vi "showLUT.vi"(0 "Palette 2":cluster{u8, u8, u8}[](array[cluster]), 1 "Palette1":cluster{u8, u8, u8}[](array[cluster])) -> ()   [LabVIEW 2013]
uses:
  <vilib>/Analysis/1siggen.llb/Ramp Pattern by Samples.vi
  <vilib>/Analysis/NI_AALBase.lvlib
panel:
  in  "LUT 2":T1(ring)=enum."cold/hot (1/4)"
  in  "LUT1":T1(ring)=enum."cold/hot (1/4)"
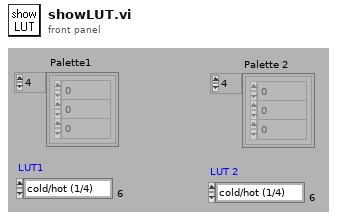
[diagram p1: front panel]
types:
  T1 = enum16{"gray", "gray + high", "gray + bounds", "gradient", "temperature", "cold/hot (1/2)", "cold/hot (1/4)", "odd/even"}
  T2 = enum32{"8 bits", "16 bits", "Float", "Complex", "RGB Chunky", "Compressed"}
  T3 = typedef "IMAQ Image.ctl" = refnum<image>
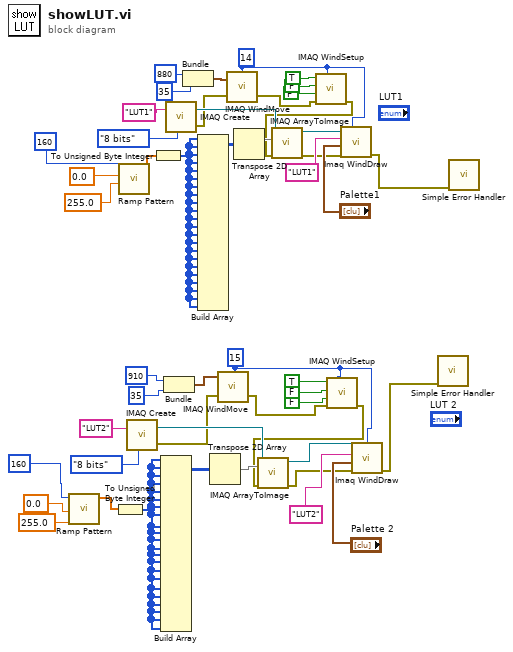
[diagram p0: block diagram]
diagram:
  w26 = 15 ("Window Number (0...15)")
  w35 = 14 ("Window Number (0...15)")
  n1 = call-poly <vilib>:"Ramp Pattern.vi"("start"=255.0, "end"=0.0, "samples"=160) -> ("Ramp Pattern"=w19:dbl[])  [unwired: 7 in, 1 out]
  n2 = To Unsigned Byte Integer(number=w19) -> (unsigned 8bit integer=w15:u8[])
  n3 = call-poly <vilib>:"Ramp Pattern.vi"("start"=255.0, "end"=0.0, "samples"=160) -> ("Ramp Pattern"=w50:dbl[])  [unwired: 7 in, 1 out]
  n4 = call "IMAQ Create"("Image Name"="LUT2", "Image Type"=T2."8 bits") -> ("New Image"=w24:T3, "error out"=w10:errorcluster)  [unwired: 2 in, 1 out]
  n5 = To Unsigned Byte Integer(number=w50) -> (unsigned 8bit integer=w34:u8[])
  n6 = Build Array(w15, w15, w15, w15, w15, w15, w15, w15, w15, w15, w15, w15, w15, w15, w15, w15, w15, w15, w15, w15, w15, w15) -> (w22:u8[][])
  n7 = Bundle(910, 35) -> (w30:cluster{i32, i32})  [unwired: 1 out]
  n8 = call "IMAQ Create"("Image Name"="LUT1", "Image Type"=T2."8 bits") -> ("New Image"=w49:T3, "error out"=w6:errorcluster)  [unwired: 2 in, 1 out]
  n9 = Bundle(880, 35) -> (w45:cluster{i32, i32})  [unwired: 1 out]
  n10 = Build Array(w34, w34, w34, w34, w34, w34, w34, w34, w34, w34, w34, w34, w34, w34, w34, w34, w34, w34, w34, w34, w34, w34) -> (w37:u8[][])
  n11 = Transpose 2D Array(2D array=w22) -> (transposed array=w23:u8[][])
  n12 = call "IMAQ WindMove"("Window Number (0...15)"=w26, "Coordinates (screen)"=w30, "error in (no error)"=w10) -> ("error out"=w9:errorcluster)  [unwired: 1 in, 2 out]
  n13 = call "IMAQ WindMove"("Window Number (0...15)"=w35, "Coordinates (screen)"=w45, "error in (no error)"=w6) -> ("error out"=w5:errorcluster)  [unwired: 1 in, 2 out]
  n14 = Transpose 2D Array(2D array=w37) -> (transposed array=w39:u8[][])
  n15 = call "IMAQ WindSetup"("Window Number (0...15)"=w35, "error in (no error)"=w5, "Window has title bar? (Yes)"=FALSE, "Window can close? (Yes)"=FALSE, "Window can grow? (Yes)"=TRUE) -> ("error out"=w4:errorcluster)  [unwired: 2 in, 4 out]
  n16 = call "IMAQ ArrayToImage"("error in (no error)"=w4, "Image Pixels (U8)"=w39, "Image"=w49) -> ("error out"=w3:errorcluster, "Image Out"=w44:T3)  [unwired: 3 in, 4 out]
  n17 = call "IMAQ WindSetup"("Window Number (0...15)"=w26, "error in (no error)"=w9, "Window has title bar? (Yes)"=FALSE ("Window can close? (Yes)"), "Window can close? (Yes)"=FALSE, "Window can grow? (Yes)"=TRUE) -> ("error out"=w8:errorcluster)  [unwired: 2 in, 4 out]
  n18 = call "IMAQ ArrayToImage"("error in (no error)"=w8, "Image Pixels (U8)"=w23, "Image"=w24) -> ("error out"=w7:errorcluster, "Image Out"=w18:T3)  [unwired: 3 in, 4 out]
  n19 = call "Imaq WindDraw"("Window Number (0...15)"=w35, "error in (no error)"=w3, "Color Palette"="Palette1", "Title"="LUT1", "Image"=w44) -> ("error out"=w2:errorcluster)  [unwired: 1 in, 5 out]
  n20 = call "Imaq WindDraw"("Window Number (0...15)"=w26, "error in (no error)"=w7, "Color Palette"="Palette 2", "Title"="LUT2", "Image"=w18) -> ("error out"=w1:errorcluster)  [unwired: 1 in, 5 out]
  n21 = call <vilib>:"Simple Error Handler.vi"("error in (no error)"=w1) -> ()  [unwired: 1 in, 8 out]
  n22 = call <vilib>:"Simple Error Handler.vi"("error in (no error)"=w2) -> ()  [unwired: 1 in, 8 out]
